vi "Autonomous Independent.vi"   [LabVIEW 2019]
doc: "This VI is called when autonomous begins, and will automatically be terminated when autonomous ends. You can carry out timed or sensor driven robot movement independently without needing to return to the caller."
uses:
  <vilib>/Rock Robotics/WPI/ThirdParty/REV Robotics/SPARK MAX/Typedef/Spark MAX Control Type.ctl
  <vilib>/Rock Robotics/WPI/Utilities/WPI_GetSetVariantRefNum.vi
  <vilib>/Rock Robotics/Network Tables/NT Read String.vi
  <vilib>/Rock Robotics/Network Tables/NT Write Numeric Array.vi
  Robot Global Data.vi
  <vilib>/Rock Robotics/Network Tables/NT Write Number.vi
  <vilib>/Rock Robotics/Network Tables/NT Read Number.vi
  <vilib>/addons/control/pid/pid.llb/PID (DBL).vi
  <vilib>/addons/control/pid/NI_PID_pid.lvlib
panel:
  # "Be sure to right-click and choose Data Operations>>Make Current Value default if you want to save the array values with the VI"
types:
  T1 = typedef "WPI_JoystickDevRef.ctl" = cluster{"Device":T2}
  T2 = typedef "WPI_JoystickDeviceEnum.ctl" = enum16{"USB 0", "USB 1", "USB 2", "USB 3", "USB 4", "USB 5"}
  T3 = typedef "WPI_ServoDeviceRef.ctl" = cluster{"DeviceStatus":errorcluster, "PWM Channel":T4, "DeadBand":T5}
  T4 = typedef "FPGA_DIOPWMChannel.ctl" = enum8{"PWM 0", "PWM 1", "PWM 2", "PWM 3", "PWM 4", "PWM 5", "PWM 6", "PWM 7", "PWM 8", "PWM 9", "PWM MXP 0", "PWM MXP 1", "PWM MXP 2", "PWM MXP 3", "PWM MXP 4", "PWM MXP 5", "PWM MXP 6", "PWM MXP 7", "PWM MXP 8", "PWM MXP 9", "Invalid"}
  T5 = typedef "WPI_PWMDeadband.ctl" = cluster{"Name":string, "maxPositivePwm":i32, "minPositivePwm":i32, "centerPwm":i32, "maxNegativePwm":i32, "minNegativePwm":i32, "angularRange":u16}
  T6 = typedef "WPI_MotorControlDeviceRef.ctl" = cluster{"DeviceStatus":errorcluster, "Type":T7, "PWM":cluster{"PWM Channel":T4, "DeadBand":T5}, "CAN":cluster{"Device Number":u8, "SetOutput VI Ref":variant, "GetOutput VI Ref":variant, "Enable VI Ref":variant, "Disable VI Ref":variant, "Data":variant}, "Invert":bool, "DIO PWM":cluster{"PWM \"Enable\" Channel":T4, "DIOChannel":T8, "PWM Rate":dbl}}
  T7 = typedef "WPI_MotorControlType.ctl" = enum16{"PWM", "CAN", "DIO PWM"}
  T8 = typedef "FPGA_DIOChannel.ctl" = enum8{"DIO 0", "DIO 1", "DIO 2", "DIO 3", "DIO 4", "DIO 5", "DIO 6", "DIO 7", "DIO 8", "DIO 9", "DIO MXP 0", "DIO MXP 1", "DIO MXP 2", "DIO MXP 3", "DIO MXP 4", "DIO MXP 5", "DIO MXP 6", "DIO MXP 7", "DIO MXP 8", "DIO MXP 9", "DIO MXP 10", "DIO MXP 11", "DIO MXP 12", "DIO MXP 13", "DIO MXP 14", "DIO MXP 15", "SPI Port CS1", "SPI Port CS2", "SPI Port CS3", "SPI Port MISO", "SPI Port MOSI", "Invalid"}
  T9 = cluster{"MotorControlDevRef":T6, "MotorControlDevRef":T6, "ServoDeviceRef":T3, "MotorControlDevRef":T6, "Distance":dbl}
  T10 = cluster{"proportional gain (Kc)":dbl, "integral time (Ti, min)":dbl, "derivative time (Td, min)":dbl}
  T11 = cluster{"P Gain":dbl, "I Gain":dbl, "D Gain":dbl, "F Gain":dbl, "I Zone":dbl, "Min Output":dbl, "Max Output":dbl}
  T12 = typedef "Spark MAX Control Type.ctl" = enum16{"Percent VBus", "Voltage", "Velocity", "Position", "Smart Motion", "Current", "Smart Velocity"}
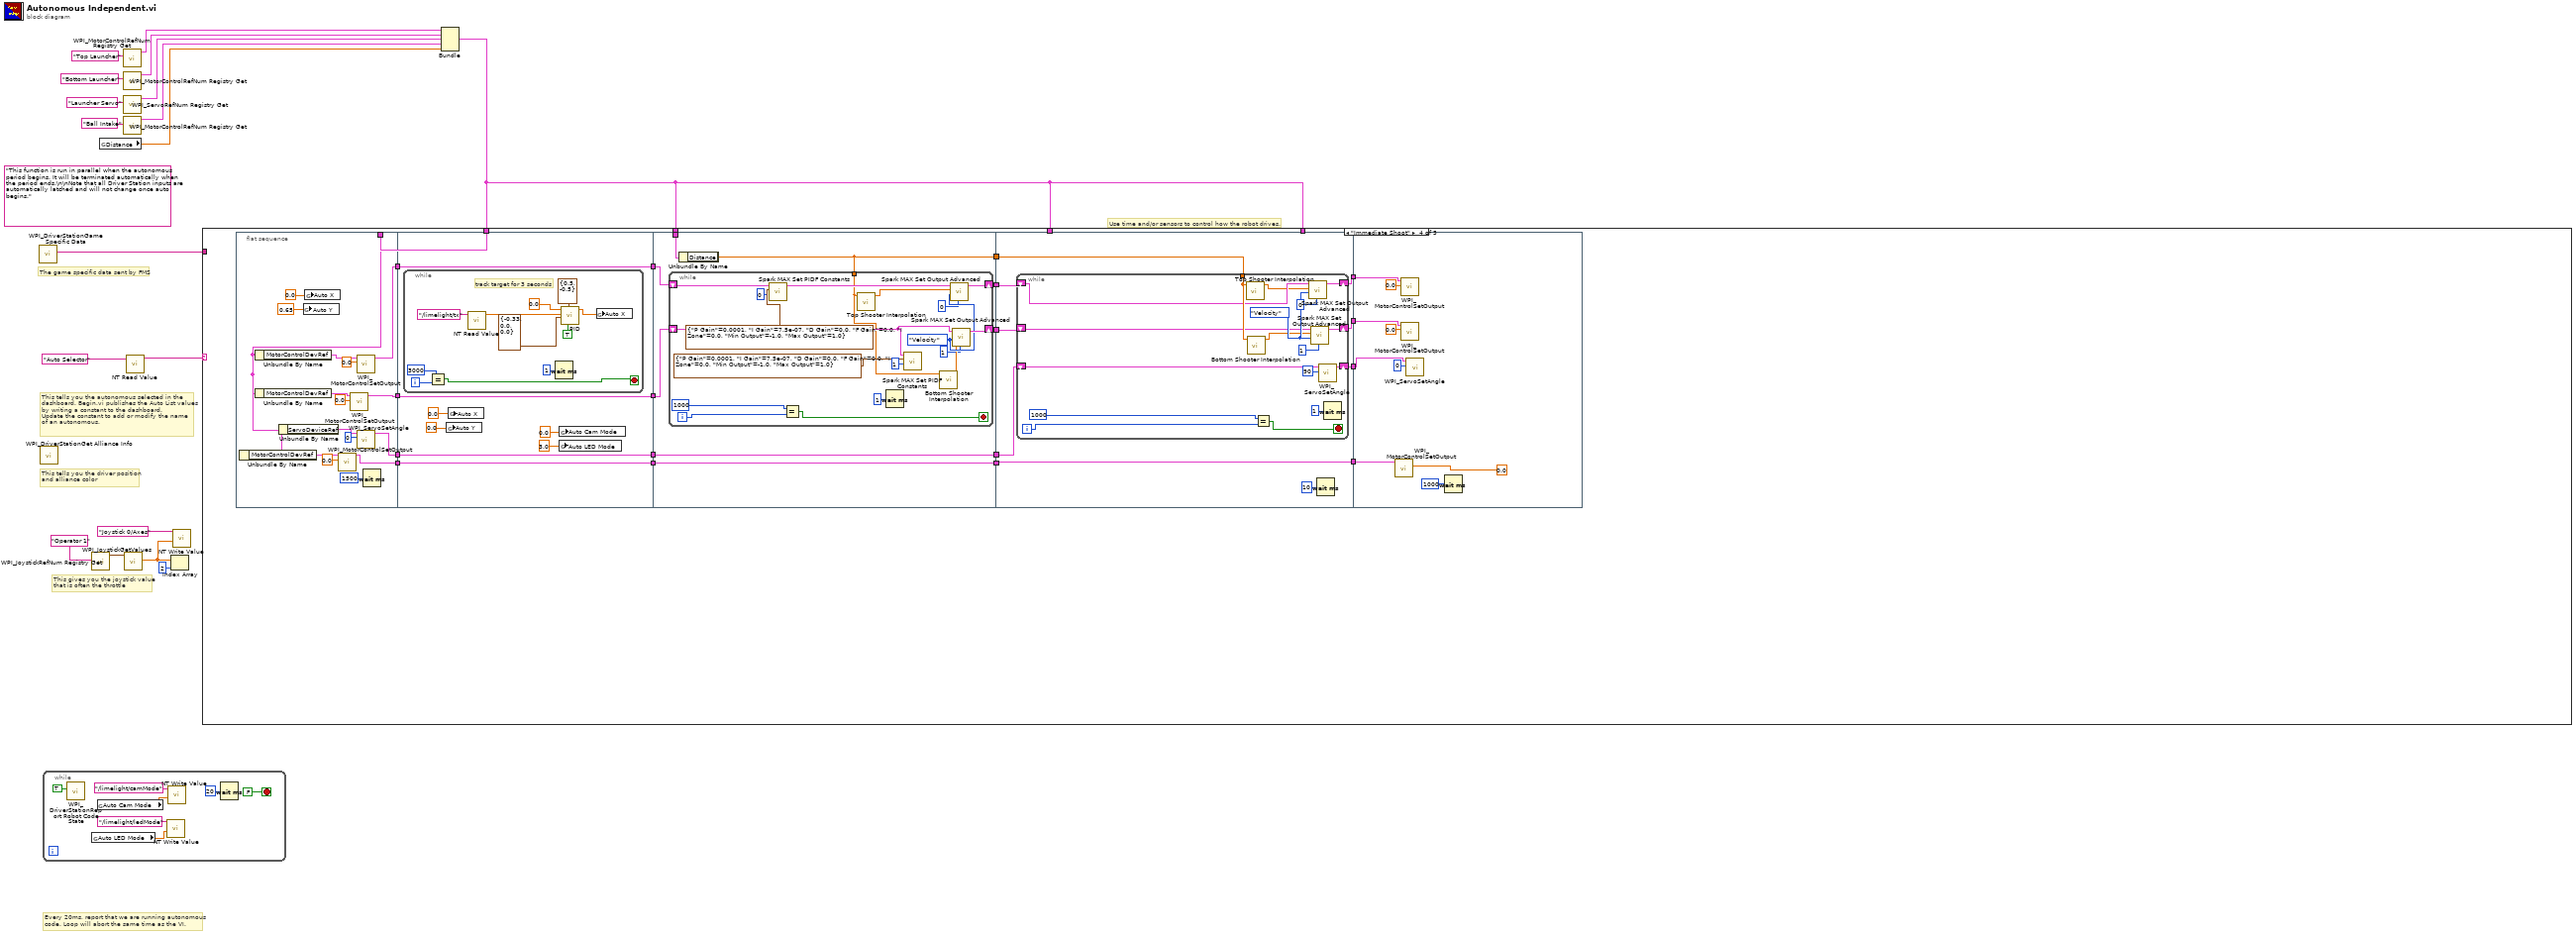
[diagram p0: block diagram]
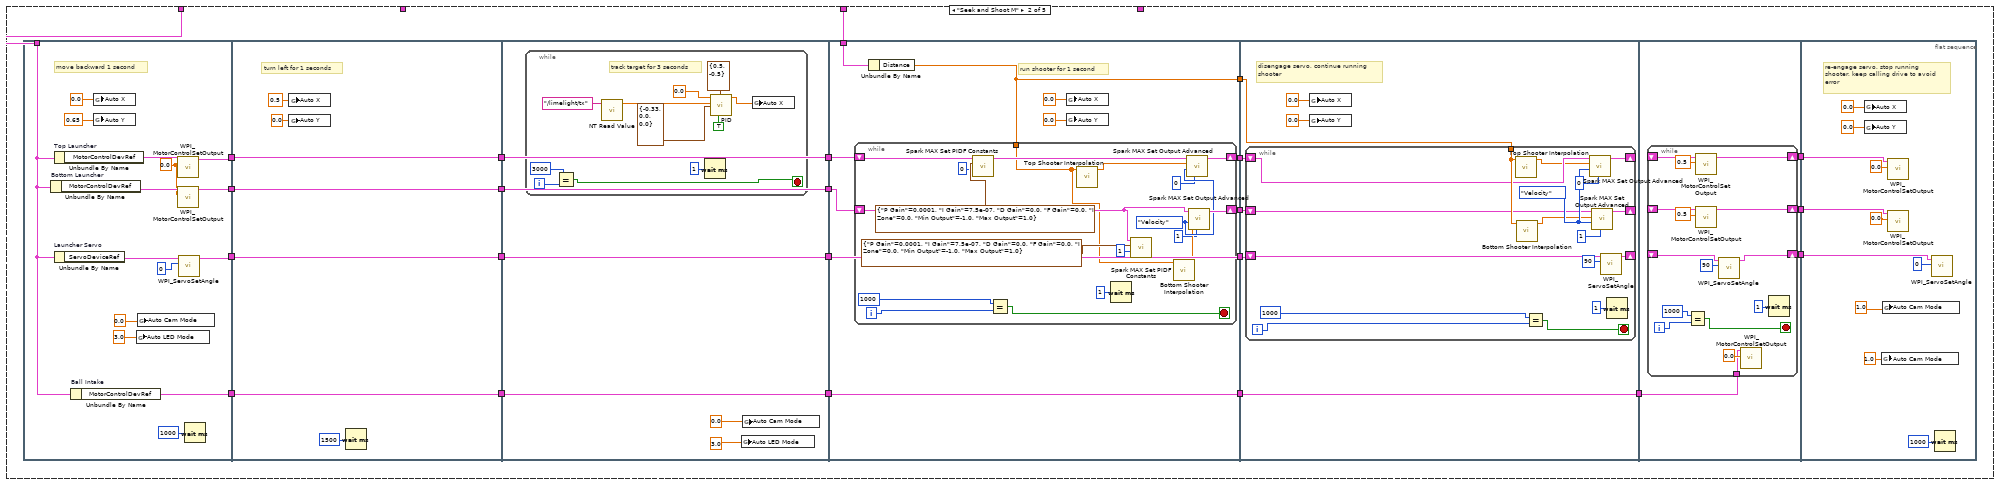
[diagram p3: hidden frame]
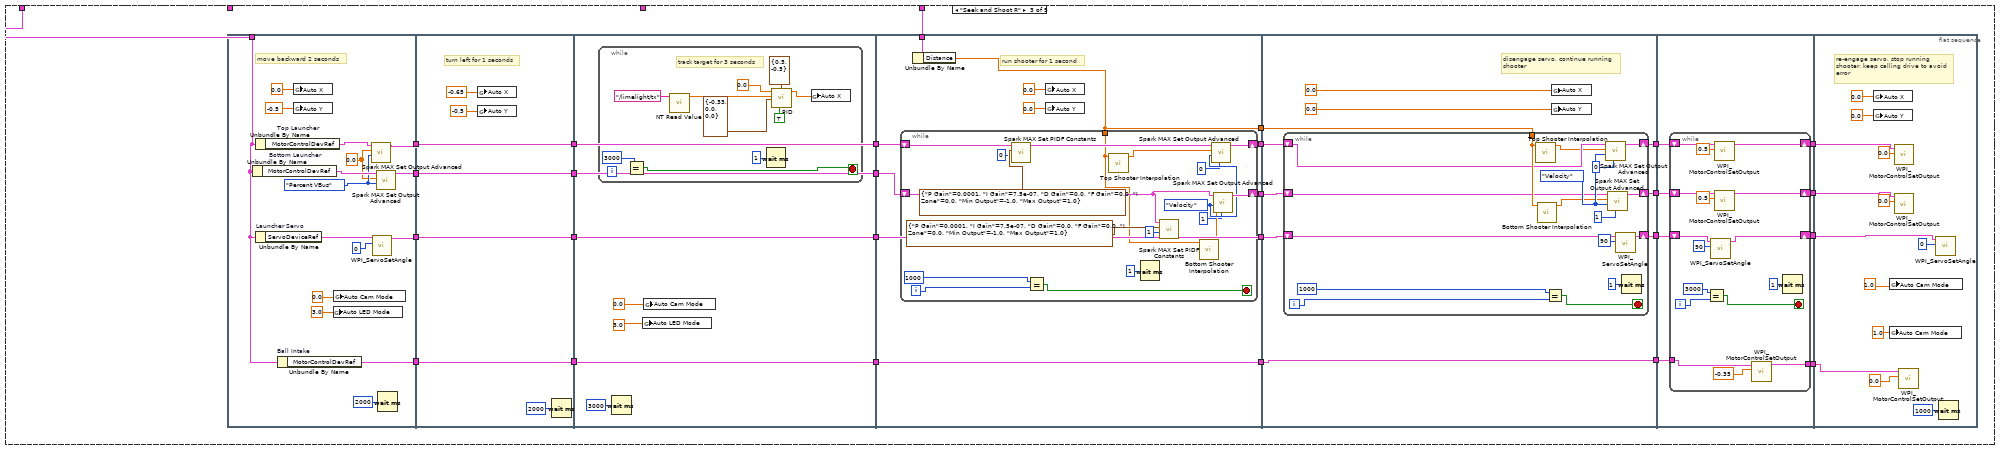
[diagram p4: hidden frame]
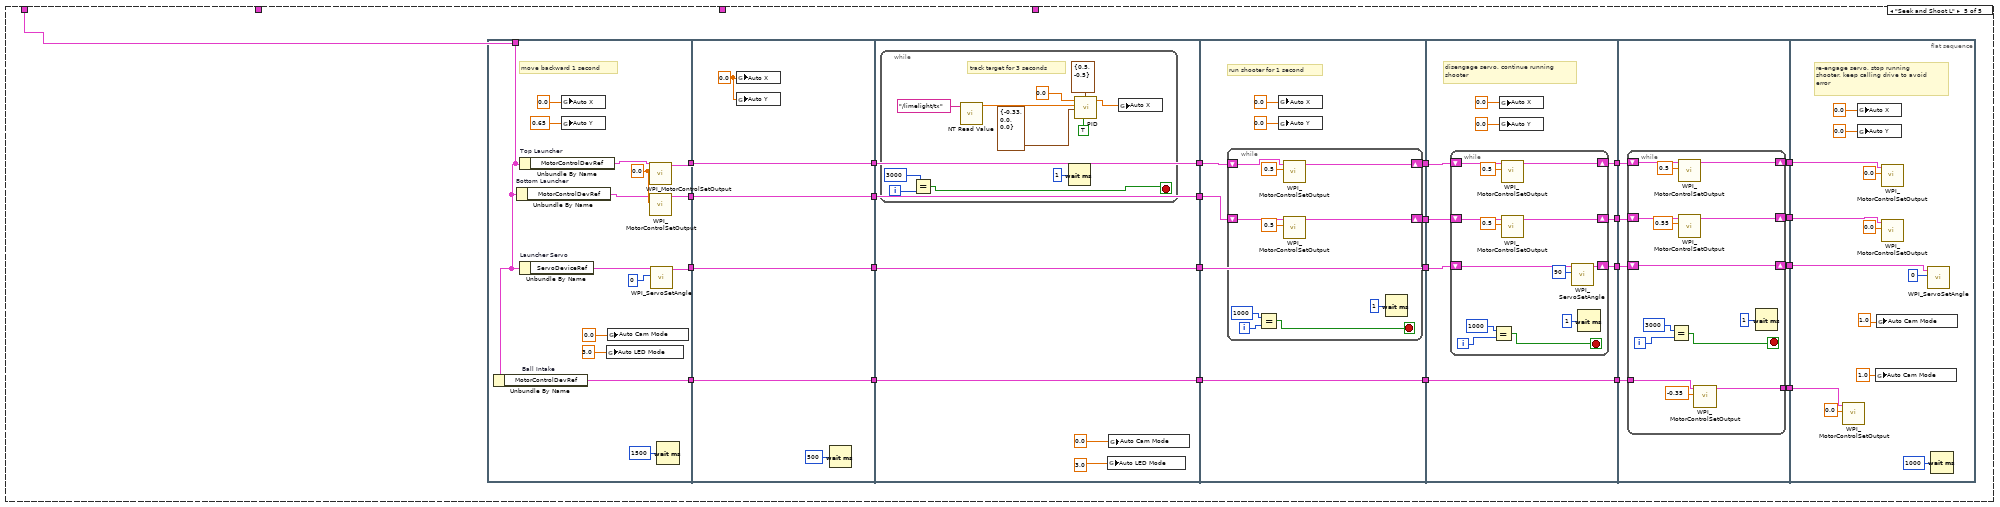
[diagram p5: hidden frame]
diagram:
  (unwired) "This function is run in parallel when the autonomous period begins. It will be terminated automatically when the period ends.\n\nNote that all Driver Station inputs are automatically latched and will not change once auto begins."
  # "The game specific data sent by FMS"
  # "This tells you the autonomous selected in the \ndashboard. Begin.vi publishes the Auto List values\nby writing a constant to the dashboard.\nUpdate the constant to add or modify the name\nof an autonomous."
  # "Every 20ms, report that we are running autonomous\ncode. Loop will abort the same time as the VI."
  # "This gives you the joystick value\nthat is often the throttle"
  # "Use time and/or sensors to control how the robot drives."
  # "This tells you the driver position\nand alliance color"
  n1 = call <vilib>:"WPI_DriverStationGame Specific Data.vi"() -> ("Game Specific Data"=w11:string)  [unwired: 11 in]
  n2 = call <vilib>:"WPI_DriverStationGet Alliance Info.vi"() -> ()  [unwired: 12 out]
  n3 = while {
    stop <- FALSE stop-if-true
    n4 = call <vilib>:"WPI_DriverStationReport Robot Code State.vi"("Autonomous"=TRUE) -> ()  [unwired: 10 in, 1 out]
    n5 = global read "Robot Global Data.vi" "Auto LED Mode"() -> (w20:dbl)
    n6 = global read "Robot Global Data.vi" "Auto Cam Mode"() -> (w19:dbl)
    n7 = call-poly <vilib>:"NT Write Value.vi"("Numeric"=w20, "Name"="/limelight/ledMode") -> ()  [unwired: 9 in, 1 out]
    n8 = call-poly <vilib>:"NT Write Value.vi"("Numeric"=w19, "Name"="/limelight/camMode") -> ()  [unwired: 9 in, 1 out]
    n9 = Wait (ms)(milliseconds to wait=u32 20) -> ()  [unwired: 1 out]
  }
  n10 = call <vilib>:"WPI_JoystickRefNum Registry Get.vi"("refnum name"="Operator 1") -> ("JoystickDevRef"=w17:T1)  [unwired: 1 in, 9 out]
  n11 = global read "Robot Global Data.vi" "Distance"() -> (w2:dbl)
  n12 = call <vilib>:"WPI_ServoRefNum Registry Get.vi"("refnum name"="Launcher Servo") -> ("ServoDeviceRef"=w5:T3)  [unwired: 9 in, 1 out]
  n13 = call <vilib>:"WPI_MotorControlRefNum Registry Get.vi"("refnum name"="Ball Intake") -> ("MotorControlDevRef"=w4:T6)  [unwired: 9 in, 1 out]
  n14 = call <vilib>:"WPI_MotorControlRefNum Registry Get.vi"("refnum name"="Top Launcher") -> ("MotorControlDevRef"=w8:T6)  [unwired: 9 in, 1 out]
  n15 = call <vilib>:"WPI_MotorControlRefNum Registry Get.vi"("refnum name"="Bottom Launcher") -> ("MotorControlDevRef"=w7:T6)  [unwired: 9 in, 1 out]
  n16 = call <vilib>:"WPI_JoystickGetValues.vi"("JoystickDevRef"=w17) -> ("Axes"=w13:dbl[])  [unwired: 6 in, 4 out]
  n17 = call-poly <vilib>:"NT Read Value.vi"("Name"="Auto Selector") -> ("String"=w14:string)  [unwired: 9 in, 1 out]
  n18 = Index Array(array=w13, index=2) -> ()  [unwired: 1 out]
  n19 = call-poly <vilib>:"NT Write Value.vi"("Numeric Array"=w13, "Name"="Joystick 0/Axes") -> ()  [unwired: 9 in, 1 out]
  n20 = Bundle("MotorControlDevRef"=w8, "MotorControlDevRef"=w7, "ServoDeviceRef"=w5, "MotorControlDevRef"=w4, "Distance"=w2) -> (w1:T9)  [unwired: 1 in]
  n21 = case shown="\"Immediate Shoot\"" w14 {
    tunnel: w11 -> [_ _ _ _ _]
    tunnel: w1 -> [_ w38 w185 w350 w460]
    tunnel: w1 -> [_ _ w172 _ _]
    tunnel: w1 -> [_ _ _ w337 _]
    tunnel: w1 -> [_ w28 _ _ _]
    frame Default {
      # "You can put your main auto here, or you can right-click on the case and make any\nother frame be the default case."
      # "This is the frame that will execute if no selection is made, or if it is not recognized"
    }
    frame "Seek and Shoot M" {
      n22 = flat-sequence {
        tunnel: w38 -> [w50]
        tunnel: [w59] -> w48
        tunnel: [w56] -> w47
        tunnel: [w53] -> w46
        tunnel: [w49] -> w37
        tunnel: [w70] -> w45
        tunnel: [w69] -> w44
        tunnel: [w68] -> w43
        tunnel: w46 -> [w68]
        tunnel: w47 -> [w70]
        tunnel: w48 -> [w69]
        tunnel: w37 -> [w64]
        tunnel: [w64] -> w36
        tunnel: w45 -> [w76]
        tunnel: [w76] -> w42
        tunnel: w44 -> [w75]
        tunnel: [w75] -> w41
        tunnel: w43 -> [w74]
        tunnel: [w74] -> w40
        tunnel: w36 -> [w71]
        tunnel: [w71] -> w35
        tunnel: w42 -> [w97]
        tunnel: w41 -> [w93]
        tunnel: [w97] -> w39
        tunnel: w40 -> [w92]
        tunnel: w35 -> [w94]
        tunnel: [w94] -> w34
        tunnel: [w91] -> w30
        tunnel: [w90] -> w29
        tunnel: w28 -> [w89]
        tunnel: [w88] -> w27
        tunnel: w39 -> [w119]
        tunnel: w34 -> [w117]
        tunnel: w30 -> [w120]
        tunnel: w29 -> [w121]
        tunnel: w27 -> [w118]
        tunnel: [w117] -> w26
        tunnel: [w144] -> w33
        tunnel: [w143] -> w32
        tunnel: [w142] -> w31
        tunnel: w26 -> [w141]
        tunnel: w33 -> [w162]
        tunnel: w32 -> [w161]
        tunnel: w31 -> [w160]
        frame #0 {
          w57 = 0.0 ("Output")
          # "move backward 1 second"
          n23 = Unbundle By Name "Bottom Launcher"(w50) -> ("MotorControlDevRef"=w58:T6)
          n24 = Unbundle By Name "Top Launcher"(w50) -> ("MotorControlDevRef"=w60:T6)
          n25 = Unbundle By Name "Launcher Servo"(w50) -> ("ServoDeviceRef"=w55:T3)
          n26 = Unbundle By Name "Ball Intake"(w50) -> ("MotorControlDevRef"=w49:T6)
          n27 = global write "Robot Global Data.vi" "Auto X"(0.0 ("Joystick X")) -> ()
          n28 = global write "Robot Global Data.vi" "Auto Y"(0.65 ("Joystick Y")) -> ()
          n29 = global write "Robot Global Data.vi" "Auto LED Mode"(3.0 ("Numeric")) -> ()
          n30 = global write "Robot Global Data.vi" "Auto Cam Mode"(0.0 ("Numeric")) -> ()
          n31 = call <vilib>:"WPI_MotorControlSetOutput.vi"("Output"=w57, "MotorControlDevRef"=w60) -> ("MotorControlDevRef"=w59:T6)  [unwired: 7 in, 2 out]
          n32 = call <vilib>:"WPI_MotorControlSetOutput.vi"("Output"=w57, "MotorControlDevRef"=w58) -> ("MotorControlDevRef"=w53:T6)  [unwired: 7 in, 2 out]
          n33 = call <vilib>:"WPI_ServoSetAngle.vi"("Angle"=0, "ServoDeviceRef"=w55) -> ("ServoDeviceRef"=w56:T3)  [unwired: 8 in, 1 out]
          n34 = Wait (ms)(milliseconds to wait=u32 1000) -> ()  [unwired: 1 out]
        }
        frame #1 {
          # "turn left for 1 seconds"
          n35 = global write "Robot Global Data.vi" "Auto X"(0.5 ("Auto X")) -> ()
          n36 = global write "Robot Global Data.vi" "Auto Y"(0.0 ("Auto Y")) -> ()
          n37 = Wait (ms)(milliseconds to wait=u32 1500) -> ()  [unwired: 1 out]
        }
        frame #2 {
          n38 = while {
            i -> [w79]
            stop <- w77 stop-if-true
            # "track target for 3 seconds"
            n39 = Equal?(x=3000, y=w79) -> (x = y?=w77:bool)
            n40 = call-poly <vilib>:"NT Read Value.vi"("Name"="/limelight/tx") -> ("Numeric"=w82:dbl)  [unwired: 9 in, 1 out]
            n41 = Wait (ms)(milliseconds to wait=u32 1) -> ()  [unwired: 1 out]
            n42 = call-poly <vilib>:"PID.vi"("reinitialize? (F)"=TRUE, "output range"=cluster{"output high":dbl, "output low":dbl} {"output high"=0.5, "output low"=-0.5}, "PID gains"=T10 {"proportional gain (Kc)"=-0.33, "integral time (Ti, min)"=0.0, "derivative time (Td, min)"=0.0}, "process variable"=w82, "setpoint"=0.0) -> ("output"=w87:dbl)  [unwired: 5 in, 1 out]
            n43 = global write "Robot Global Data.vi" "Auto X"(w87) -> ()
          }
          n44 = global write "Robot Global Data.vi" "Auto LED Mode"(3.0 ("Numeric")) -> ()
          n45 = global write "Robot Global Data.vi" "Auto Cam Mode"(0.0 ("Numeric")) -> ()
        }
        frame #3 {
          # "run shooter for 1 second"
          n46 = Unbundle By Name(w89) -> ("Distance"=w88:dbl)
          n47 = while {
            shift-right: [w107] -> w90
            shift-left: w93 -> [w108]
            shift-right: [w106] -> w91
            shift-left: w92 -> [w105]
            tunnel: w88 -> [w99]
            i -> [w115]
            stop <- w113 stop-if-true
            w103 = Spark_MAX_Control_Type."Velocity" ("Control Mode")
            n48 = call <vilib>:"Spark MAX Set PIDF Constants.vi"("PIDF Slot"=0, "PID Constants"=T11 {"P Gain"=0.0001, "I Gain"=7.5e-07, "D Gain"=0.0, "F Gain"=0.0, "I Zone"=0.0, "Min Output"=-1.0, "Max Output"=1.0}, "MotorControlDeviceRef"=w108) -> ("MotorControlDeviceRef"=w104:T6)  [unwired: 7 in, 1 out]
            n49 = Equal?(x=1000 ("y"), y=w115) -> (x = y?=w113:bool)
            n50 = call "Top Shooter Interpolation.vi"("Distance"=w99) -> ("interpolation value"=w102:dbl)  [unwired: 10 in]
            n51 = Wait (ms)(milliseconds to wait=u32 1) -> ()  [unwired: 1 out]
            n52 = call <vilib>:"Spark MAX Set PIDF Constants.vi"("PIDF Slot"=1, "PID Constants"=T11 {"P Gain"=0.0001, "I Gain"=7.5e-07, "D Gain"=0.0, "F Gain"=0.0, "I Zone"=0.0, "Min Output"=-1.0, "Max Output"=1.0}, "MotorControlDeviceRef"=w105) -> ()  [unwired: 7 in, 2 out]
            n53 = call "Bottom Shooter Interpolation.vi"("Distance"=w99) -> ("interpolation value"=w101:dbl)  [unwired: 10 in]
            n54 = call <vilib>:"Spark MAX Set Output Advanced.vi"("PIDF Slot (0)"=0, "Control Mode"=w103, "Setpoint"=w102, "MotorControlDevRef"=w104) -> ("MotorControlDevRef"=w107:T6)  [unwired: 6 in, 1 out]
            n55 = call <vilib>:"Spark MAX Set Output Advanced.vi"("PIDF Slot (0)"=1, "Control Mode"=w103, "Setpoint"=w101, "MotorControlDevRef"=w105) -> ("MotorControlDevRef"=w106:T6)  [unwired: 6 in, 1 out]
          }
          n56 = global write "Robot Global Data.vi" "Auto X"(0.0 ("Joystick X")) -> ()
          n57 = global write "Robot Global Data.vi" "Auto Y"(0.0 ("Joystick Y")) -> ()
        }
        frame #4 {
          # "disengage servo, continue running\nshooter"
          n58 = while {
            shift-right: [w133] -> _
            shift-left: w121 -> [w126]
            shift-right: [w132] -> _
            shift-left: w120 -> [w125]
            shift-right: [w139] -> _
            shift-left: w119 -> [w140]
            tunnel: w118 -> [w130]
            i -> [w135]
            stop <- w134 stop-if-true
            w131 = Spark_MAX_Control_Type."Velocity" ("Control Mode")
            n59 = call "Top Shooter Interpolation.vi"("Distance"=w130) -> ("interpolation value"=w124:dbl)  [unwired: 10 in]
            n60 = call "Bottom Shooter Interpolation.vi"("Distance"=w130) -> ("interpolation value"=w129:dbl)  [unwired: 10 in]
            n61 = Equal?(x=1000 ("y"), y=w135) -> (x = y?=w134:bool)
            n62 = call <vilib>:"Spark MAX Set Output Advanced.vi"("PIDF Slot (0)"=0, "Control Mode"=w131, "Setpoint"=w124, "MotorControlDevRef"=w126) -> ("MotorControlDevRef"=w133:T6)  [unwired: 6 in, 1 out]
            n63 = call <vilib>:"Spark MAX Set Output Advanced.vi"("PIDF Slot (0)"=1, "Control Mode"=w131, "Setpoint"=w129, "MotorControlDevRef"=w125) -> ("MotorControlDevRef"=w132:T6)  [unwired: 6 in, 1 out]
            n64 = call <vilib>:"WPI_ServoSetAngle.vi"("Angle"=90, "ServoDeviceRef"=w140) -> ("ServoDeviceRef"=w139:T3)  [unwired: 8 in, 1 out]
            n65 = Wait (ms)(milliseconds to wait=u32 1) -> ()  [unwired: 1 out]
          }
          n66 = global write "Robot Global Data.vi" "Auto X"(0.0 ("Joystick X")) -> ()
          n67 = global write "Robot Global Data.vi" "Auto Y"(0.0 ("Joystick Y")) -> ()
        }
        frame #5 {
          n68 = while {
            shift-right: [w156] -> w142
            shift-left: _ -> [w159]
            shift-right: [w157] -> w143
            shift-left: _ -> [w158]
            shift-right: [w146] -> w144
            shift-left: _ -> [w147]
            tunnel: w141 -> [w145]
            i -> [w151]
            stop <- w150 stop-if-true
            n69 = Equal?(x=1000 ("y"), y=w151) -> (x = y?=w150:bool)
            n70 = call <vilib>:"WPI_MotorControlSetOutput.vi"("Output"=0.5, "MotorControlDevRef"=w159) -> ("MotorControlDevRef"=w156:T6)  [unwired: 7 in, 2 out]
            n71 = call <vilib>:"WPI_MotorControlSetOutput.vi"("Output"=0.5, "MotorControlDevRef"=w158) -> ("MotorControlDevRef"=w157:T6)  [unwired: 7 in, 2 out]
            n72 = call <vilib>:"WPI_ServoSetAngle.vi"("Angle"=90, "ServoDeviceRef"=w147) -> ("ServoDeviceRef"=w146:T3)  [unwired: 8 in, 1 out]
            n73 = call <vilib>:"WPI_MotorControlSetOutput.vi"("Output"=0.0, "MotorControlDevRef"=w145) -> ()  [unwired: 7 in, 3 out]
            n74 = Wait (ms)(milliseconds to wait=u32 1) -> ()  [unwired: 1 out]
          }
        }
        frame #6 {
          # "re-engage servo, stop running\nshooter, keep calling drive to avoid\nerror"
          n75 = global write "Robot Global Data.vi" "Auto X"(0.0 ("Joystick X")) -> ()
          n76 = global write "Robot Global Data.vi" "Auto Y"(0.0 ("Joystick Y")) -> ()
          n77 = global write "Robot Global Data.vi" "Auto Cam Mode"(1.0 ("Numeric")) -> ()
          n78 = global write "Robot Global Data.vi" "Auto Cam Mode"(1.0 ("Numeric")) -> ()
          n79 = call <vilib>:"WPI_MotorControlSetOutput.vi"("Output"=0.0, "MotorControlDevRef"=w160) -> ()  [unwired: 7 in, 3 out]
          n80 = call <vilib>:"WPI_MotorControlSetOutput.vi"("Output"=0.0, "MotorControlDevRef"=w161) -> ()  [unwired: 7 in, 3 out]
          n81 = call <vilib>:"WPI_ServoSetAngle.vi"("Angle"=0, "ServoDeviceRef"=w162) -> ()  [unwired: 8 in, 2 out]
          n82 = Wait (ms)(milliseconds to wait=u32 1000) -> ()  [unwired: 1 out]
        }
      }
    }
    frame "Seek and Shoot R" {
      n83 = flat-sequence {
        tunnel: [w203] -> w197
        tunnel: [w210] -> w196
        tunnel: [w201] -> w195
        tunnel: w185 -> [w205]
        tunnel: [w204] -> w181
        tunnel: w197 -> [w219]
        tunnel: w196 -> [w220]
        tunnel: [w220] -> w194
        tunnel: [w219] -> w193
        tunnel: w195 -> [w215]
        tunnel: [w215] -> w192
        tunnel: w181 -> [w214]
        tunnel: [w214] -> w180
        tunnel: [w227] -> w191
        tunnel: [w226] -> w190
        tunnel: [w225] -> w189
        tunnel: [w222] -> w179
        tunnel: w194 -> [w227]
        tunnel: w193 -> [w226]
        tunnel: w192 -> [w225]
        tunnel: w180 -> [w222]
        tunnel: w191 -> [w245]
        tunnel: w190 -> [w248]
        tunnel: [w247] -> w188
        tunnel: [w246] -> w187
        tunnel: [w245] -> w186
        tunnel: w189 -> [w242]
        tunnel: w179 -> [w241]
        tunnel: [w241] -> w178
        tunnel: w172 -> [w240]
        tunnel: [w239] -> w171
        tunnel: w188 -> [w277]
        tunnel: w187 -> [w276]
        tunnel: w186 -> [w275]
        tunnel: [w274] -> w184
        tunnel: [w273] -> w183
        tunnel: [w272] -> w182
        tunnel: w178 -> [w269]
        tunnel: [w269] -> w177
        tunnel: w171 -> [w268]
        tunnel: w184 -> [w300]
        tunnel: w183 -> [w301]
        tunnel: w182 -> [w302]
        tunnel: w177 -> [w299]
        tunnel: [w298] -> w176
        tunnel: [w297] -> w175
        tunnel: [w296] -> w174
        tunnel: [w295] -> w173
        tunnel: w176 -> [w322]
        tunnel: w175 -> [w321]
        tunnel: w174 -> [w320]
        tunnel: w173 -> [w319]
        frame #0 {
          w199 = Spark_MAX_Control_Type."Percent VBus" ("Control Mode")
          w198 = 0.0 ("Output")
          # "move backward 2 seconds"
          n84 = Unbundle By Name "Bottom Launcher"(w205) -> ("MotorControlDevRef"=w200:T6)
          n85 = Unbundle By Name "Top Launcher"(w205) -> ("MotorControlDevRef"=w202:T6)
          n86 = Unbundle By Name "Launcher Servo"(w205) -> ("ServoDeviceRef"=w206:T3)
          n87 = Unbundle By Name "Ball Intake"(w205) -> ("MotorControlDevRef"=w204:T6)
          n88 = global write "Robot Global Data.vi" "Auto X"(0.0 ("Joystick X")) -> ()
          n89 = global write "Robot Global Data.vi" "Auto Y"(-0.5 ("Joystick Y")) -> ()
          n90 = global write "Robot Global Data.vi" "Auto LED Mode"(3.0 ("Numeric")) -> ()
          n91 = global write "Robot Global Data.vi" "Auto Cam Mode"(0.0 ("Numeric")) -> ()
          n92 = call <vilib>:"Spark MAX Set Output Advanced.vi"("Control Mode"=w199, "Setpoint"=w198, "MotorControlDevRef"=w202) -> ("MotorControlDevRef"=w203:T6)  [unwired: 7 in, 1 out]
          n93 = call <vilib>:"WPI_ServoSetAngle.vi"("Angle"=0, "ServoDeviceRef"=w206) -> ("ServoDeviceRef"=w210:T3)  [unwired: 8 in, 1 out]
          n94 = call <vilib>:"Spark MAX Set Output Advanced.vi"("Control Mode"=w199, "Setpoint"=w198, "MotorControlDevRef"=w200) -> ("MotorControlDevRef"=w201:T6)  [unwired: 7 in, 1 out]
          n95 = Wait (ms)(milliseconds to wait=u32 2000) -> ()  [unwired: 1 out]
        }
        frame #1 {
          # "turn left for 1 seconds"
          n96 = global write "Robot Global Data.vi" "Auto X"(-0.65 ("Joystick X")) -> ()
          n97 = global write "Robot Global Data.vi" "Auto Y"(-0.5 ("Joystick Y")) -> ()
          n98 = Wait (ms)(milliseconds to wait=u32 2000) -> ()  [unwired: 1 out]
        }
        frame #2 {
          n99 = while {
            i -> [w230]
            stop <- w228 stop-if-true
            # "track target for 3 seconds"
            n100 = Equal?(x=3000, y=w230) -> (x = y?=w228:bool)
            n101 = call-poly <vilib>:"NT Read Value.vi"("Name"="/limelight/tx") -> ("Numeric"=w233:dbl)  [unwired: 9 in, 1 out]
            n102 = Wait (ms)(milliseconds to wait=u32 1) -> ()  [unwired: 1 out]
            n103 = call-poly <vilib>:"PID.vi"("reinitialize? (F)"=TRUE, "output range"=cluster{"output high":dbl, "output low":dbl} {"output high"=0.5, "output low"=-0.5}, "PID gains"=T10 {"proportional gain (Kc)"=-0.33, "integral time (Ti, min)"=0.0, "derivative time (Td, min)"=0.0}, "process variable"=w233, "setpoint"=0.0) -> ("output"=w238:dbl)  [unwired: 5 in, 1 out]
            n104 = global write "Robot Global Data.vi" "Auto X"(w238) -> ()
          }
          n105 = Wait (ms)(milliseconds to wait=u32 3000) -> ()  [unwired: 1 out]
          n106 = global write "Robot Global Data.vi" "Auto LED Mode"(3.0 ("Numeric")) -> ()
          n107 = global write "Robot Global Data.vi" "Auto Cam Mode"(0.0 ("Numeric")) -> ()
        }
        frame #3 {
          # "run shooter for 1 second"
          n108 = Unbundle By Name(w240) -> ("Distance"=w239:dbl)
          n109 = while {
            shift-right: [w258] -> w247
            shift-left: w248 -> [w259]
            shift-right: [w257] -> w246
            shift-left: w242 -> [w256]
            tunnel: w239 -> [w252]
            i -> [w266]
            stop <- w264 stop-if-true
            w254 = Spark_MAX_Control_Type."Velocity" ("Control Mode")
            n110 = call <vilib>:"Spark MAX Set PIDF Constants.vi"("PIDF Slot"=0, "PID Constants"=T11 {"P Gain"=0.0001, "I Gain"=7.5e-07, "D Gain"=0.0, "F Gain"=0.0, "I Zone"=0.0, "Min Output"=-1.0, "Max Output"=1.0}, "MotorControlDeviceRef"=w259) -> ("MotorControlDeviceRef"=w255:T6)  [unwired: 7 in, 1 out]
            n111 = Equal?(x=1000 ("y"), y=w266) -> (x = y?=w264:bool)
            n112 = call "Top Shooter Interpolation.vi"("Distance"=w252) -> ("interpolation value"=w253:dbl)  [unwired: 10 in]
            n113 = Wait (ms)(milliseconds to wait=u32 1) -> ()  [unwired: 1 out]
            n114 = call <vilib>:"Spark MAX Set PIDF Constants.vi"("PIDF Slot"=1, "PID Constants"=T11 {"P Gain"=0.0001, "I Gain"=7.5e-07, "D Gain"=0.0, "F Gain"=0.0, "I Zone"=0.0, "Min Output"=-1.0, "Max Output"=1.0}, "MotorControlDeviceRef"=w256) -> ()  [unwired: 7 in, 2 out]
            n115 = call "Bottom Shooter Interpolation.vi"("Distance"=w252) -> ("interpolation value"=w251:dbl)  [unwired: 10 in]
            n116 = call <vilib>:"Spark MAX Set Output Advanced.vi"("PIDF Slot (0)"=0, "Control Mode"=w254, "Setpoint"=w253, "MotorControlDevRef"=w255) -> ("MotorControlDevRef"=w258:T6)  [unwired: 6 in, 1 out]
            n117 = call <vilib>:"Spark MAX Set Output Advanced.vi"("PIDF Slot (0)"=1, "Control Mode"=w254, "Setpoint"=w251, "MotorControlDevRef"=w256) -> ("MotorControlDevRef"=w257:T6)  [unwired: 6 in, 1 out]
          }
          n118 = global write "Robot Global Data.vi" "Auto X"(0.0 ("Joystick X")) -> ()
          n119 = global write "Robot Global Data.vi" "Auto Y"(0.0 ("Joystick Y")) -> ()
        }
        frame #4 {
          # "disengage servo, continue running\nshooter"
          n120 = while {
            shift-right: [w287] -> w272
            shift-left: w277 -> [w280]
            shift-right: [w286] -> w273
            shift-left: w276 -> [w279]
            shift-right: [w293] -> w274
            shift-left: w275 -> [w294]
            tunnel: w268 -> [w284]
            i -> [w289]
            stop <- w288 stop-if-true
            w285 = Spark_MAX_Control_Type."Velocity" ("Control Mode")
            n121 = call "Top Shooter Interpolation.vi"("Distance"=w284) -> ("interpolation value"=w278:dbl)  [unwired: 10 in]
            n122 = call "Bottom Shooter Interpolation.vi"("Distance"=w284) -> ("interpolation value"=w283:dbl)  [unwired: 10 in]
            n123 = Equal?(x=1000 ("y"), y=w289) -> (x = y?=w288:bool)
            n124 = call <vilib>:"Spark MAX Set Output Advanced.vi"("PIDF Slot (0)"=0, "Control Mode"=w285, "Setpoint"=w278, "MotorControlDevRef"=w280) -> ("MotorControlDevRef"=w287:T6)  [unwired: 6 in, 1 out]
            n125 = call <vilib>:"Spark MAX Set Output Advanced.vi"("PIDF Slot (0)"=1, "Control Mode"=w285, "Setpoint"=w283, "MotorControlDevRef"=w279) -> ("MotorControlDevRef"=w286:T6)  [unwired: 6 in, 1 out]
            n126 = call <vilib>:"WPI_ServoSetAngle.vi"("Angle"=90, "ServoDeviceRef"=w294) -> ("ServoDeviceRef"=w293:T3)  [unwired: 8 in, 1 out]
            n127 = Wait (ms)(milliseconds to wait=u32 1) -> ()  [unwired: 1 out]
          }
          n128 = global write "Robot Global Data.vi" "Auto X"(0.0 ("Joystick X")) -> ()
          n129 = global write "Robot Global Data.vi" "Auto Y"(0.0 ("Joystick Y")) -> ()
        }
        frame #5 {
          n130 = while {
            shift-right: [w315] -> w297
            shift-left: w302 -> [w318]
            shift-right: [w316] -> w296
            shift-left: w301 -> [w317]
            shift-right: [w303] -> w295
            shift-left: w300 -> [w304]
            tunnel: [w307] -> w298
            tunnel: w299 -> [w306]
            i -> [w310]
            stop <- w309 stop-if-true
            n131 = Equal?(x=3000 ("y"), y=w310) -> (x = y?=w309:bool)
            n132 = call <vilib>:"WPI_ServoSetAngle.vi"("Angle"=90, "ServoDeviceRef"=w304) -> ("ServoDeviceRef"=w303:T3)  [unwired: 8 in, 1 out]
            n133 = call <vilib>:"WPI_MotorControlSetOutput.vi"("Output"=0.5, "MotorControlDevRef"=w318) -> ("MotorControlDevRef"=w315:T6)  [unwired: 7 in, 2 out]
            n134 = call <vilib>:"WPI_MotorControlSetOutput.vi"("Output"=0.5, "MotorControlDevRef"=w317) -> ("MotorControlDevRef"=w316:T6)  [unwired: 7 in, 2 out]
            n135 = call <vilib>:"WPI_MotorControlSetOutput.vi"("Output"=-0.35, "MotorControlDevRef"=w306) -> ("MotorControlDevRef"=w307:T6)  [unwired: 7 in, 2 out]
            n136 = Wait (ms)(milliseconds to wait=u32 1) -> ()  [unwired: 1 out]
          }
        }
        frame #6 {
          # "re-engage servo, stop running\nshooter, keep calling drive to avoid\nerror"
          n137 = global write "Robot Global Data.vi" "Auto X"(0.0 ("Joystick X")) -> ()
          n138 = global write "Robot Global Data.vi" "Auto Y"(0.0 ("Joystick Y")) -> ()
          n139 = global write "Robot Global Data.vi" "Auto Cam Mode"(1.0 ("Numeric")) -> ()
          n140 = global write "Robot Global Data.vi" "Auto Cam Mode"(1.0 ("Numeric")) -> ()
          n141 = call <vilib>:"WPI_MotorControlSetOutput.vi"("Output"=0.0, "MotorControlDevRef"=w321) -> ()  [unwired: 7 in, 3 out]
          n142 = call <vilib>:"WPI_MotorControlSetOutput.vi"("Output"=0.0, "MotorControlDevRef"=w320) -> ()  [unwired: 7 in, 3 out]
          n143 = call <vilib>:"WPI_MotorControlSetOutput.vi"("Output"=0.0, "MotorControlDevRef"=w322) -> ()  [unwired: 7 in, 3 out]
          n144 = call <vilib>:"WPI_ServoSetAngle.vi"("Angle"=0, "ServoDeviceRef"=w319) -> ()  [unwired: 8 in, 2 out]
          n145 = Wait (ms)(milliseconds to wait=u32 1000) -> ()  [unwired: 1 out]
        }
      }
    }
    frame "Immediate Shoot" {
      n146 = flat-sequence {
        tunnel: w350 -> [w363]
        tunnel: [w357] -> w348
        tunnel: [w359] -> w346
        tunnel: [w355] -> w343
        tunnel: [w361] -> w340
        tunnel: [w370] -> w349
        tunnel: w348 -> [w370]
        tunnel: [w369] -> w347
        tunnel: w346 -> [w369]
        tunnel: [w368] -> w344
        tunnel: w343 -> [w368]
        tunnel: [w367] -> w341
        tunnel: w340 -> [w367]
        tunnel: w349 -> [w391]
        tunnel: w347 -> [w390]
        tunnel: [w393] -> w345
        tunnel: w344 -> [w393]
        tunnel: [w392] -> w342
        tunnel: w341 -> [w392]
        tunnel: [w389] -> w339
        tunnel: [w388] -> w338
        tunnel: w337 -> [w387]
        tunnel: [w386] -> w336
        tunnel: w338 -> [w420]
        tunnel: w339 -> [w421]
        tunnel: w342 -> [w414]
        tunnel: w345 -> [w419]
        tunnel: w336 -> [w418]
        tunnel: [w417] -> w335
        tunnel: [w416] -> w334
        tunnel: [w415] -> w333
        tunnel: [w414] -> w332
        tunnel: w335 -> [w442]
        tunnel: w334 -> [w441]
        tunnel: w333 -> [w440]
        tunnel: w332 -> [w439]
        frame #0 {
          n147 = Unbundle By Name(w363) -> ("MotorControlDevRef"=w362:T6)
          n148 = Unbundle By Name(w363) -> ("MotorControlDevRef"=w358:T6)
          n149 = Unbundle By Name(w363) -> ("MotorControlDevRef"=w360:T6)
          n150 = Unbundle By Name(w363) -> ("ServoDeviceRef"=w356:T3)
          n151 = global write "Robot Global Data.vi" "Auto Y"(0.65 ("Joystick Y")) -> ()
          n152 = global write "Robot Global Data.vi" "Auto X"(0.0 ("Joystick X")) -> ()
          n153 = call <vilib>:"WPI_MotorControlSetOutput.vi"("Output"=0.0, "MotorControlDevRef"=w362) -> ("MotorControlDevRef"=w361:T6)  [unwired: 7 in, 2 out]
          n154 = call <vilib>:"WPI_MotorControlSetOutput.vi"("Output"=0.0, "MotorControlDevRef"=w360) -> ("MotorControlDevRef"=w359:T6)  [unwired: 7 in, 2 out]
          n155 = call <vilib>:"WPI_MotorControlSetOutput.vi"("Output"=0.0, "MotorControlDevRef"=w358) -> ("MotorControlDevRef"=w357:T6)  [unwired: 7 in, 2 out]
          n156 = call <vilib>:"WPI_ServoSetAngle.vi"("Angle"=0, "ServoDeviceRef"=w356) -> ("ServoDeviceRef"=w355:T3)  [unwired: 8 in, 1 out]
          n157 = Wait (ms)(milliseconds to wait=u32 1500) -> ()  [unwired: 1 out]
        }
        frame #1 {
          n158 = while {
            i -> [w377]
            stop <- w375 stop-if-true
            # "track target for 3 seconds"
            n159 = Equal?(x=3000, y=w377) -> (x = y?=w375:bool)
            n160 = call-poly <vilib>:"NT Read Value.vi"("Name"="/limelight/tx") -> ("Numeric"=w380:dbl)  [unwired: 9 in, 1 out]
            n161 = Wait (ms)(milliseconds to wait=u32 1) -> ()  [unwired: 1 out]
            n162 = call-poly <vilib>:"PID.vi"("reinitialize? (F)"=TRUE, "output range"=cluster{"output high":dbl, "output low":dbl} {"output high"=0.5, "output low"=-0.5}, "PID gains"=T10 {"proportional gain (Kc)"=-0.33, "integral time (Ti, min)"=0.0, "derivative time (Td, min)"=0.0}, "process variable"=w380, "setpoint"=0.0) -> ("output"=w385:dbl)  [unwired: 5 in, 1 out]
            n163 = global write "Robot Global Data.vi" "Auto X"(w385) -> ()
          }
          n164 = global write "Robot Global Data.vi" "Auto Y"(0.0 ("Joystick Y")) -> ()
          n165 = global write "Robot Global Data.vi" "Auto X"(0.0 ("Joystick X")) -> ()
          n166 = global write "Robot Global Data.vi" "Auto LED Mode"(3.0 ("Numeric")) -> ()
          n167 = global write "Robot Global Data.vi" "Auto Cam Mode"(0.0 ("Numeric")) -> ()
        }
        frame #2 {
          n168 = Unbundle By Name(w387) -> ("Distance"=w386:dbl)
          n169 = while {
            shift-right: [w403] -> w389
            shift-left: w391 -> [w404]
            shift-right: [w402] -> w388
            shift-left: w390 -> [w401]
            tunnel: w386 -> [w397]
            i -> [w411]
            stop <- w409 stop-if-true
            w399 = Spark_MAX_Control_Type."Velocity" ("Control Mode")
            n170 = call <vilib>:"Spark MAX Set PIDF Constants.vi"("PIDF Slot"=0, "PID Constants"=T11 {"P Gain"=0.0001, "I Gain"=7.5e-07, "D Gain"=0.0, "F Gain"=0.0, "I Zone"=0.0, "Min Output"=-1.0, "Max Output"=1.0}, "MotorControlDeviceRef"=w404) -> ("MotorControlDeviceRef"=w400:T6)  [unwired: 7 in, 1 out]
            n171 = Equal?(x=1000 ("y"), y=w411) -> (x = y?=w409:bool)
            n172 = call "Top Shooter Interpolation.vi"("Distance"=w397) -> ("interpolation value"=w398:dbl)  [unwired: 10 in]
            n173 = Wait (ms)(milliseconds to wait=u32 1) -> ()  [unwired: 1 out]
            n174 = call <vilib>:"Spark MAX Set PIDF Constants.vi"("PIDF Slot"=1, "PID Constants"=T11 {"P Gain"=0.0001, "I Gain"=7.5e-07, "D Gain"=0.0, "F Gain"=0.0, "I Zone"=0.0, "Min Output"=-1.0, "Max Output"=1.0}, "MotorControlDeviceRef"=w401) -> ()  [unwired: 7 in, 2 out]
            n175 = call "Bottom Shooter Interpolation.vi"("Distance"=w397) -> ("interpolation value"=w396:dbl)  [unwired: 10 in]
            n176 = call <vilib>:"Spark MAX Set Output Advanced.vi"("PIDF Slot (0)"=0, "Control Mode"=w399, "Setpoint"=w398, "MotorControlDevRef"=w400) -> ("MotorControlDevRef"=w403:T6)  [unwired: 6 in, 1 out]
            n177 = call <vilib>:"Spark MAX Set Output Advanced.vi"("PIDF Slot (0)"=1, "Control Mode"=w399, "Setpoint"=w396, "MotorControlDevRef"=w401) -> ("MotorControlDevRef"=w402:T6)  [unwired: 6 in, 1 out]
          }
        }
        frame #3 {
          n178 = while {
            shift-right: [w431] -> w415
            shift-left: w421 -> [w424]
            shift-right: [w430] -> w416
            shift-left: w420 -> [w423]
            shift-right: [w437] -> w417
            shift-left: w419 -> [w438]
            tunnel: w418 -> [w428]
            i -> [w433]
            stop <- w432 stop-if-true
            w429 = Spark_MAX_Control_Type."Velocity" ("Control Mode")
            n179 = call "Top Shooter Interpolation.vi"("Distance"=w428) -> ("interpolation value"=w422:dbl)  [unwired: 10 in]
            n180 = call "Bottom Shooter Interpolation.vi"("Distance"=w428) -> ("interpolation value"=w427:dbl)  [unwired: 10 in]
            n181 = Equal?(x=1000 ("y"), y=w433) -> (x = y?=w432:bool)
            n182 = call <vilib>:"Spark MAX Set Output Advanced.vi"("PIDF Slot (0)"=0, "Control Mode"=w429, "Setpoint"=w422, "MotorControlDevRef"=w424) -> ("MotorControlDevRef"=w431:T6)  [unwired: 6 in, 1 out]
            n183 = call <vilib>:"Spark MAX Set Output Advanced.vi"("PIDF Slot (0)"=1, "Control Mode"=w429, "Setpoint"=w427, "MotorControlDevRef"=w423) -> ("MotorControlDevRef"=w430:T6)  [unwired: 6 in, 1 out]
            n184 = call <vilib>:"WPI_ServoSetAngle.vi"("Angle"=90, "ServoDeviceRef"=w438) -> ("ServoDeviceRef"=w437:T3)  [unwired: 8 in, 1 out]
            n185 = Wait (ms)(milliseconds to wait=u32 1) -> ()  [unwired: 1 out]
          }
          n186 = Wait (ms)(milliseconds to wait=u32 10) -> ()  [unwired: 1 out]
        }
        frame #4 {
          n187 = call <vilib>:"WPI_MotorControlSetOutput.vi"("Output"=0.0, "MotorControlDevRef"=w439) -> ()  [unwired: 7 in, 3 out]
          n188 = call <vilib>:"WPI_MotorControlSetOutput.vi"("Output"=0.0, "MotorControlDevRef"=w440) -> ()  [unwired: 7 in, 3 out]
          n189 = call <vilib>:"WPI_MotorControlSetOutput.vi"("Output"=0.0, "MotorControlDevRef"=w441) -> ()  [unwired: 7 in, 3 out]
          n190 = call <vilib>:"WPI_ServoSetAngle.vi"("Angle"=0, "ServoDeviceRef"=w442) -> ()  [unwired: 8 in, 2 out]
          n191 = Wait (ms)(milliseconds to wait=u32 1000) -> ()  [unwired: 1 out]
        }
      }
    }
    frame "Seek and Shoot L" {
      n192 = flat-sequence {
        tunnel: [w484] -> w472
        tunnel: [w482] -> w471
        tunnel: [w480] -> w470
        tunnel: w460 -> [w474]
        tunnel: [w473] -> w456
        tunnel: [w493] -> w469
        tunnel: [w492] -> w468
        tunnel: [w491] -> w467
        tunnel: w470 -> [w491]
        tunnel: w471 -> [w493]
        tunnel: w472 -> [w492]
        tunnel: w456 -> [w488]
        tunnel: [w488] -> w455
        tunnel: w469 -> [w499]
        tunnel: [w499] -> w466
        tunnel: w468 -> [w498]
        tunnel: [w498] -> w465
        tunnel: w467 -> [w497]
        tunnel: [w497] -> w464
        tunnel: w455 -> [w494]
        tunnel: [w494] -> w454
        tunnel: w466 -> [w515]
        tunnel: w465 -> [w518]
        tunnel: [w517] -> w463
        tunnel: [w516] -> w462
        tunnel: [w515] -> w461
        tunnel: w464 -> [w512]
        tunnel: w454 -> [w511]
        tunnel: [w511] -> w453
        tunnel: w463 -> [w537]
        tunnel: w462 -> [w536]
        tunnel: w461 -> [w535]
        tunnel: [w534] -> w459
        tunnel: [w533] -> w458
        tunnel: [w532] -> w457
        tunnel: w453 -> [w529]
        tunnel: [w529] -> w452
        tunnel: w459 -> [w556]
        tunnel: w458 -> [w557]
        tunnel: w457 -> [w558]
        tunnel: w452 -> [w555]
        tunnel: [w554] -> w451
        tunnel: [w553] -> w450
        tunnel: [w552] -> w449
        tunnel: [w551] -> w448
        tunnel: w451 -> [w576]
        tunnel: w450 -> [w575]
        tunnel: w449 -> [w574]
        tunnel: w448 -> [w573]
        frame #0 {
          w483 = 0.0 ("Output")
          # "move backward 1 second"
          n193 = Unbundle By Name "Ball Intake"(w474) -> ("MotorControlDevRef"=w473:T6)
          n194 = Unbundle By Name "Bottom Launcher"(w474) -> ("MotorControlDevRef"=w476:T6)
          n195 = Unbundle By Name "Top Launcher"(w474) -> ("MotorControlDevRef"=w477:T6)
          n196 = Unbundle By Name "Launcher Servo"(w474) -> ("ServoDeviceRef"=w475:T3)
          n197 = global write "Robot Global Data.vi" "Auto X"(0.0 ("Joystick X")) -> ()
          n198 = global write "Robot Global Data.vi" "Auto Y"(0.65 ("Joystick Y")) -> ()
          n199 = global write "Robot Global Data.vi" "Auto LED Mode"(3.0 ("Numeric")) -> ()
          n200 = global write "Robot Global Data.vi" "Auto Cam Mode"(0.0 ("Numeric")) -> ()
          n201 = call <vilib>:"WPI_MotorControlSetOutput.vi"("Output"=w483, "MotorControlDevRef"=w477) -> ("MotorControlDevRef"=w484:T6)  [unwired: 7 in, 2 out]
          n202 = call <vilib>:"WPI_MotorControlSetOutput.vi"("Output"=w483, "MotorControlDevRef"=w476) -> ("MotorControlDevRef"=w480:T6)  [unwired: 7 in, 2 out]
          n203 = call <vilib>:"WPI_ServoSetAngle.vi"("Angle"=0, "ServoDeviceRef"=w475) -> ("ServoDeviceRef"=w482:T3)  [unwired: 8 in, 1 out]
          n204 = Wait (ms)(milliseconds to wait=u32 1500) -> ()  [unwired: 1 out]
        }
        frame #1 {
          w489 = 0.0 ("Auto X")
          n205 = global write "Robot Global Data.vi" "Auto X"(w489) -> ()
          n206 = global write "Robot Global Data.vi" "Auto Y"(w489) -> ()
          n207 = Wait (ms)(milliseconds to wait=u32 500) -> ()  [unwired: 1 out]
        }
        frame #2 {
          n208 = while {
            i -> [w502]
            stop <- w500 stop-if-true
            # "track target for 3 seconds"
            n209 = Equal?(x=3000, y=w502) -> (x = y?=w500:bool)
            n210 = call-poly <vilib>:"NT Read Value.vi"("Name"="/limelight/tx") -> ("Numeric"=w505:dbl)  [unwired: 9 in, 1 out]
            n211 = Wait (ms)(milliseconds to wait=u32 1) -> ()  [unwired: 1 out]
            n212 = call-poly <vilib>:"PID.vi"("reinitialize? (F)"=TRUE, "output range"=cluster{"output high":dbl, "output low":dbl} {"output high"=0.5, "output low"=-0.5}, "PID gains"=T10 {"proportional gain (Kc)"=-0.33, "integral time (Ti, min)"=0.0, "derivative time (Td, min)"=0.0}, "process variable"=w505, "setpoint"=0.0) -> ("output"=w510:dbl)  [unwired: 5 in, 1 out]
            n213 = global write "Robot Global Data.vi" "Auto X"(w510) -> ()
          }
          n214 = global write "Robot Global Data.vi" "Auto LED Mode"(3.0 ("Numeric")) -> ()
          n215 = global write "Robot Global Data.vi" "Auto Cam Mode"(0.0 ("Numeric")) -> ()
        }
        frame #3 {
          # "run shooter for 1 second"
          n216 = while {
            shift-right: [w527] -> w517
            shift-left: w518 -> [w528]
            shift-right: [w526] -> w516
            shift-left: w512 -> [w523]
            i -> [w521]
            stop <- w519 stop-if-true
            n217 = Equal?(x=1000 ("y"), y=w521) -> (x = y?=w519:bool)
            n218 = call <vilib>:"WPI_MotorControlSetOutput.vi"("Output"=0.5, "MotorControlDevRef"=w528) -> ("MotorControlDevRef"=w527:T6)  [unwired: 7 in, 2 out]
            n219 = call <vilib>:"WPI_MotorControlSetOutput.vi"("Output"=0.5, "MotorControlDevRef"=w523) -> ("MotorControlDevRef"=w526:T6)  [unwired: 7 in, 2 out]
            n220 = Wait (ms)(milliseconds to wait=u32 1) -> ()  [unwired: 1 out]
          }
          n221 = global write "Robot Global Data.vi" "Auto X"(0.0 ("Joystick X")) -> ()
          n222 = global write "Robot Global Data.vi" "Auto Y"(0.0 ("Joystick Y")) -> ()
        }
        frame #4 {
          # "disengage servo, continue running\nshooter"
          n223 = while {
            shift-right: [w545] -> w532
            shift-left: w537 -> [w550]
            shift-right: [w546] -> w533
            shift-left: w536 -> [w549]
            shift-right: [w547] -> w534
            shift-left: w535 -> [w548]
            i -> [w539]
            stop <- w538 stop-if-true
            n224 = Equal?(x=1000 ("y"), y=w539) -> (x = y?=w538:bool)
            n225 = call <vilib>:"WPI_MotorControlSetOutput.vi"("Output"=0.5, "MotorControlDevRef"=w550) -> ("MotorControlDevRef"=w545:T6)  [unwired: 7 in, 2 out]
            n226 = call <vilib>:"WPI_MotorControlSetOutput.vi"("Output"=0.5, "MotorControlDevRef"=w549) -> ("MotorControlDevRef"=w546:T6)  [unwired: 7 in, 2 out]
            n227 = call <vilib>:"WPI_ServoSetAngle.vi"("Angle"=90, "ServoDeviceRef"=w548) -> ("ServoDeviceRef"=w547:T3)  [unwired: 8 in, 1 out]
            n228 = Wait (ms)(milliseconds to wait=u32 1) -> ()  [unwired: 1 out]
          }
          n229 = global write "Robot Global Data.vi" "Auto X"(0.0 ("Joystick X")) -> ()
          n230 = global write "Robot Global Data.vi" "Auto Y"(0.0 ("Joystick Y")) -> ()
        }
        frame #5 {
          n231 = while {
            shift-right: [w569] -> w553
            shift-left: w558 -> [w572]
            shift-right: [w570] -> w552
            shift-left: w557 -> [w571]
            shift-right: [w560] -> w551
            shift-left: w556 -> [w560]
            tunnel: w555 -> [w562]
            tunnel: [w561] -> w554
            i -> [w565]
            stop <- w564 stop-if-true
            n232 = Equal?(x=3000 ("y"), y=w565) -> (x = y?=w564:bool)
            n233 = call <vilib>:"WPI_MotorControlSetOutput.vi"("Output"=0.5, "MotorControlDevRef"=w572) -> ("MotorControlDevRef"=w569:T6)  [unwired: 7 in, 2 out]
            n234 = call <vilib>:"WPI_MotorControlSetOutput.vi"("Output"=0.55, "MotorControlDevRef"=w571) -> ("MotorControlDevRef"=w570:T6)  [unwired: 7 in, 2 out]
            n235 = call <vilib>:"WPI_MotorControlSetOutput.vi"("Output"=-0.35, "MotorControlDevRef"=w562) -> ("MotorControlDevRef"=w561:T6)  [unwired: 7 in, 2 out]
            n236 = Wait (ms)(milliseconds to wait=u32 1) -> ()  [unwired: 1 out]
          }
        }
        frame #6 {
          # "re-engage servo, stop running\nshooter, keep calling drive to avoid\nerror"
          n237 = call <vilib>:"WPI_MotorControlSetOutput.vi"("Output"=0.0, "MotorControlDevRef"=w576) -> ()  [unwired: 7 in, 3 out]
          n238 = global write "Robot Global Data.vi" "Auto X"(0.0 ("Joystick X")) -> ()
          n239 = global write "Robot Global Data.vi" "Auto Y"(0.0 ("Joystick Y")) -> ()
          n240 = global write "Robot Global Data.vi" "Auto Cam Mode"(1.0 ("Numeric")) -> ()
          n241 = global write "Robot Global Data.vi" "Auto Cam Mode"(1.0 ("Numeric")) -> ()
          n242 = call <vilib>:"WPI_MotorControlSetOutput.vi"("Output"=0.0, "MotorControlDevRef"=w575) -> ()  [unwired: 7 in, 3 out]
          n243 = call <vilib>:"WPI_MotorControlSetOutput.vi"("Output"=0.0, "MotorControlDevRef"=w574) -> ()  [unwired: 7 in, 3 out]
          n244 = call <vilib>:"WPI_ServoSetAngle.vi"("Angle"=0, "ServoDeviceRef"=w573) -> ()  [unwired: 8 in, 2 out]
          n245 = Wait (ms)(milliseconds to wait=u32 1000) -> ()  [unwired: 1 out]
        }
      }
    }
  }
